vi "MDPtr DAQ Example.vi"() -> ()   [LabVIEW 2017]
uses:
  <vilib>/Utility/Data Type/Type Definitions/Data Type.ctl
  MDPtr TypeDef/MDPtr.ctl
  54395307-d518-4202-990a-94b812b105bc.vi
  9cd2cd57-26eb-46a0-897a-d177a379a7ae.vi
  4b70eac3-4565-41a8-8678-ce1595016193.vi
  <vilib>/Utility/High Resolution Relative Seconds.vi
  <vilib>/Utility/Data Type/Get Type Information.vi
  _Support/_MDPtr Validate DataFrame Type.vi
  _PolymorphicVIs/MDPtr Unpack Memory.vi
  Advanced/MDPtr DecrementCount.vi
  _PolymorphicVIs/MDPtr Pack Memory.vi
  MDPtr.lvlib
  <vilib>/measure/NI_MABase.lvlib
  _MDPtrMgr/MDPtrMgr.lvclass
  <vilib>/Utility/Data Type/NI_Data Type.lvlib
panel:
  out "time esliped?":dbl
  in  "milliseconds to wait 2":u32=1
  out "Value out":i64
  out "Queue Names":string[](array[string])
  out "time diff(s) 3":dbl
  out "time diff(s) 2":dbl
  out "time diff(s)":dbl
  in  "Fs":dbl=1000.0 format="%#_13g"
  out "# free elements in queue":i32
  out "# elements in queue":i32
  out "#queues":i32
  out "File Logging?":bool
  out "MDPtr Total Count":i64
  in  "file path":path=path "D:/MDPtr.tdms"
  out "Square":waveform(dbl)(graph)
  out "Sine":waveform(dbl)(graph)
  in  "stop":bool
  out "Copy Count":i32
  out "Common.Data Type":T1
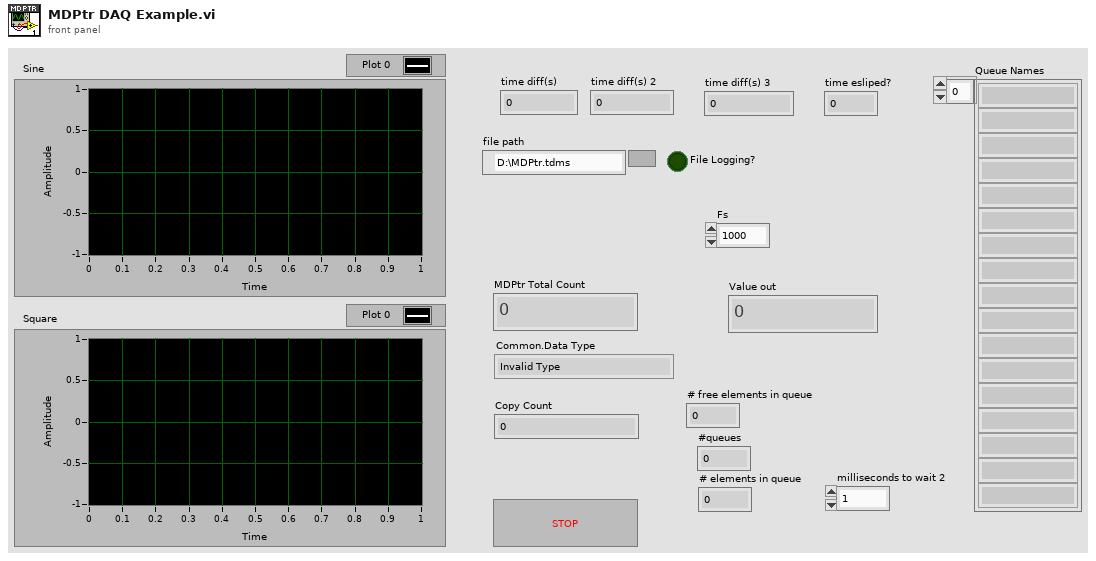
[diagram p1: front panel]
types:
  T1 = typedef "NI_Data Type.lvlib/Data Type.ctl" = enum8{"Invalid Type", "Void", "I8", "I16", "I32", "I64", "U8", "U16", "U32", "U64", "Single Float", "Double Float", "Extended Float", "Single Complex", "Double Complex", "Extended Complex", "Enum U8", "Enum U16", "Enum U32", "Enum U64", "Single Float With Unit", "Double Float With Unit", "Extended Float With Unit", "Single Complex with Unit", "Double Complex with Unit", "Extended Complex with Unit", "Boolean", "String", "Path", "Picture", "Tag", "Array", "Cluster", "Variant", "LV Variant", "Waveform", "Timestamp", "Digital Waveform", "Digital Data", "ExpressData", "Refnum", "External Data", "VI", "Poly VI", "LabVIEW Class Instance", "Fixed Point"}
  T2 = enum16{"open", "open or create", "create or replace", "create", "open (read-only)"}
  T3 = typedef "MDPtr.lvlib/MDPtr.ctl" = refnum<k1>
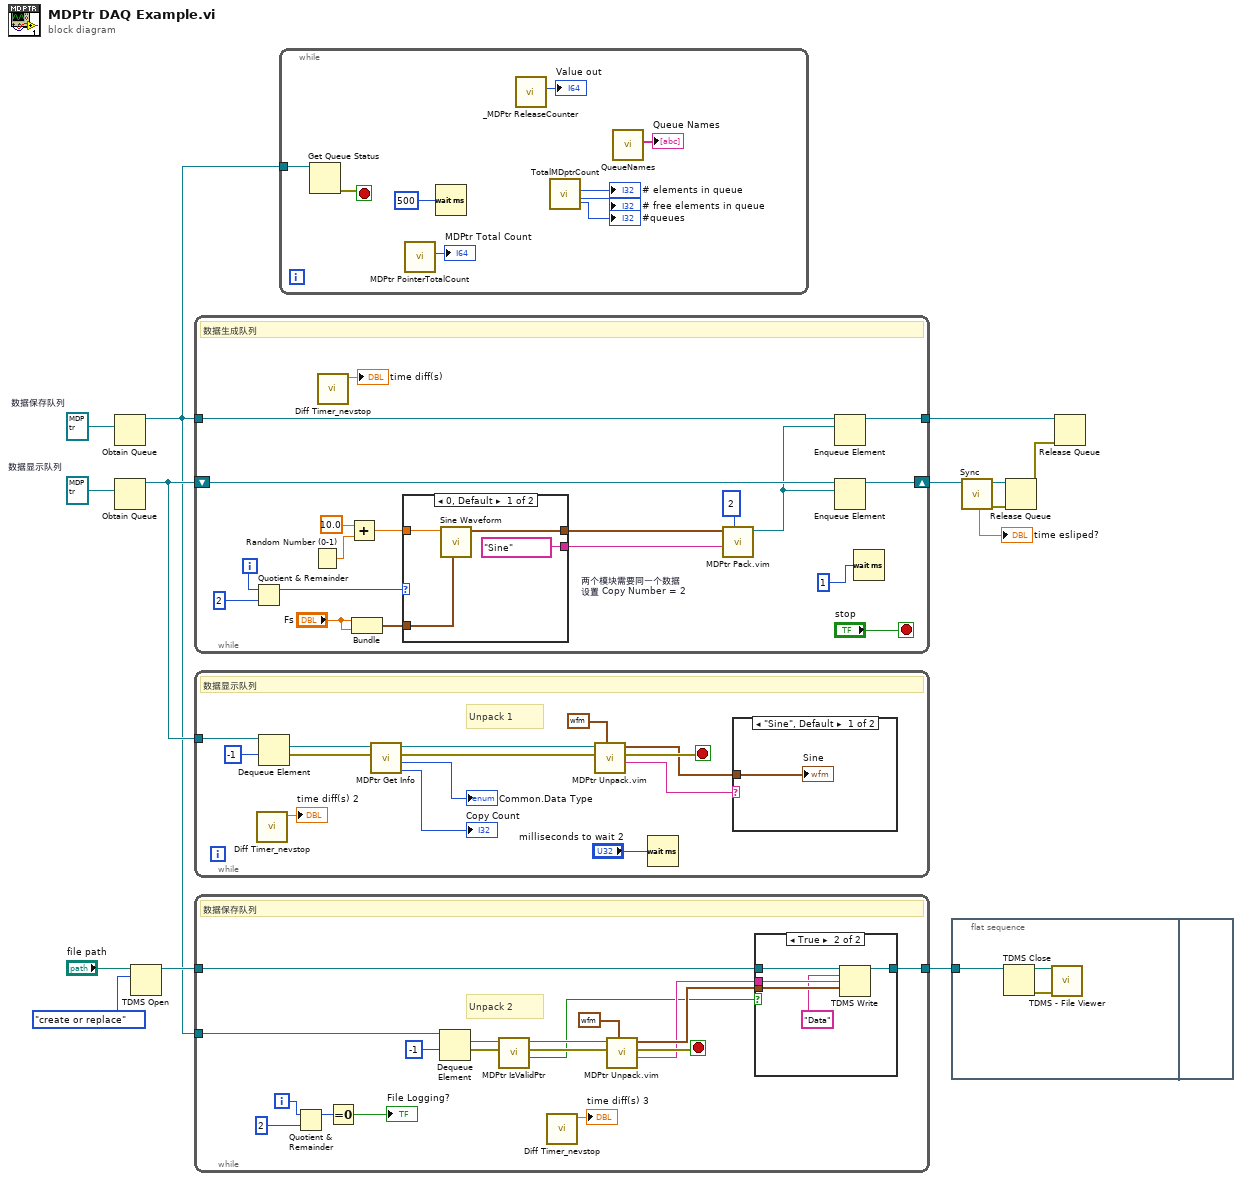
[diagram p0: block diagram]
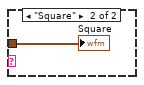
[diagram p3: hidden frame]
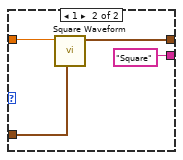
[diagram p4: hidden frame]
diagram:
  n1 = Obtain Queue "数据保存队列"(element data type=T3 refnum ("MDPtr")) -> (queue out=w4:refnum<queue>)  [unwired: 4 in, 2 out]
  n2 = Obtain Queue "数据显示队列"(element data type=T3 refnum ("MDPtr")) -> (queue out=w10:refnum<queue>)  [unwired: 4 in, 2 out]
  n3 = TDMS Open(10:T2."create or replace" ("operation (0:open)"), 11:"file path") -> (3:w8:refnum<k34>)  [unwired: 5 in, 1 out]
  n4 = while {
    shift-right: [w31] -> w5
    shift-left: w10 -> [w32]
    tunnel: w4 -> [w20]
    tunnel: [w19] -> w6
    i -> [w29]
    stop <- "stop" stop-if-true
    w21 = 2  # 两个模块需要同一个数据 设置 Copy Number = 2
    # "数据生成队列"
    n5 = Quotient & Remainder(x=w29, y=2) -> (x-y*floor(x/y)=w27:i32)  [unwired: 1 out]
    n6 = Random Number (0-1)() -> (number: 0 to 1=w23:dbl)
    n7 = call <userlib>:"Diff Timer_nevstop.vi"() -> ("time diff(s)"=→"time diff(s)":dbl)  [unwired: 10 in, 1 out]
    n8 = Add(x=10.0 ("frequency"), y=w23) -> (x+y=w22:dbl)
    n9 = Bundle("Fs"="Fs", "Fs"="Fs") -> (w15:cluster{"Fs":dbl, "Fs":dbl})  [unwired: 1 in]
    n10 = case shown="0, Default" w27 {
      tunnel: [w36 w40] -> w17
      tunnel: ["Sine" ("String Attribute") "Square" ("String Attribute")] -> w26
      tunnel: w22 -> [w34 w38]
      tunnel: w15 -> [w33 w37]
      frame 0, Default {
        n11 = call <vilib>:"Sine Waveform.vi"("sampling info"=w33, "frequency"=w34) -> ("signal out"=w36:waveform(dbl))  [unwired: 8 in, 1 out]
      }
      frame 1 {
        n12 = call <vilib>:"Square Waveform.vi"("sampling info"=w37, "frequency"=w38) -> ("signal out"=w40:waveform(dbl))  [unwired: 8 in, 1 out]
      }
    }
    n13 = call "MDPtr Pack.vim"("Copies Count(1)"=w21, "String Attribute"=w26, "Data"=w17) -> ("HexStrPtr"=w18:T3)  [unwired: 7 in, 1 out]
    n14 = Enqueue Element(queue=w20, element=w18) -> (queue out=w19:refnum<queue>)  [unwired: 2 in, 2 out]
    n15 = Enqueue Element(queue=w32, element=w18) -> (queue out=w31:refnum<queue>)  [unwired: 2 in, 2 out]
    n16 = Wait (ms)(milliseconds to wait=u32 1) -> ()  [unwired: 1 out]
  }
  n17 = while {
    tunnel: w10 -> [w54]
    stop <- w52 stop-if-true
    # "Unpack 1"
    # "数据显示队列"
    n18 = call <userlib>:"Diff Timer_nevstop.vi"() -> ("time diff(s)"=→"time diff(s) 2":dbl)  [unwired: 10 in, 1 out]
    n19 = Dequeue Element(queue=w54, timeout in ms (-1)=-1) -> (element=w44:T3, error out=w50:errorcluster)  [unwired: 1 in, 2 out]
    n20 = call "MDPtr Get Info.vi"("error in (no error)"=w50, "HexStrPtr"=w44) -> ("Copy Count"=→"Copy Count":i32, "Data Type"=→"Common.Data Type":T1, "error out"=w49:errorcluster, "HexStrPtr (dup)"=w47:T3)  [unwired: 5 in, 1 out]
    n21 = call "MDPtr Unpack.vim"("Prototype"=waveform(dbl) {"t0"=timestamp(0 s since 1904-01-01), "dt"=1.0, "Y"=[]} ("Square"), "error in (no error)"=w49, "HexStrPtr"=w47) -> ("String Attribute"=w46:string, "error out"=w52:errorcluster, "Data"=w45:waveform(dbl))  [unwired: 6 in]
    n22 = Wait (ms)(milliseconds to wait="milliseconds to wait 2") -> ()  [unwired: 1 out]
    n23 = case shown="\"Sine\", Default" w46 {
      tunnel: w45 -> [w55 w56]
      frame "Sine", Default {
        "Sine" <- w55
      }
      frame "Square" {
        "Square" <- w56
      }
    }
  }
  n24 = while {
    tunnel: w4 -> [w74]
    tunnel: [w69] -> w9
    tunnel: w8 -> [w70]
    i -> [w61]
    stop <- w72 stop-if-true
    # "Unpack 2"
    # "数据保存队列"
    n25 = Quotient & Remainder(x=w61, y=2) -> (x-y*floor(x/y)=w60:i32)  [unwired: 1 out]
    n26 = Equal To 0?(x=w60) -> (x = 0?=→"File Logging?":bool)
    n27 = Dequeue Element(queue=w74, timeout in ms (-1)=-1) -> (element=w71:T3, error out=w64:errorcluster)  [unwired: 1 in, 2 out]
    n28 = call "MDPtr IsValidPtr.vi"("error in (no error)"=w64, "HexStrPtr"=w71) -> ("Valid MDPtr?"=w63:bool, "error out"=w65:errorcluster, "HexStrPtr (dup)"=w66:T3)  [unwired: 6 in]
    n29 = call <userlib>:"Diff Timer_nevstop.vi"() -> ("time diff(s)"=→"time diff(s) 3":dbl)  [unwired: 10 in, 1 out]
    n30 = call "MDPtr Unpack.vim"("Prototype"=waveform(dbl) {"t0"=timestamp(0 s since 1904-01-01), "dt"=1.0, "Y"=[]} ("Square"), "error in (no error)"=w65, "HexStrPtr"=w66) -> ("String Attribute"=w67:string, "error out"=w72:errorcluster, "Data"=w68:waveform(dbl))  [unwired: 6 in]
    n31 = case shown="True" w63 {
      tunnel: w70 -> [w75 w80]
      tunnel: [w75 w79] -> w69
      tunnel: w68 -> [_ w78]
      tunnel: w67 -> [_ w77]
      frame False {
      }
      frame True {
        n32 = TDMS Write(0:w80, 5:"Data" ("group name in (Untitled)"), 7:w77, 9:w78) -> (4:w79:refnum<k34>)  [unwired: 2 in, 3 out]
      }
    }
  }
  n33 = while {
    tunnel: w4 -> [w89]
    stop <- w88 stop-if-true
    n34 = Get Queue Status(queue=w89) -> (error out=w88:errorcluster)  [unwired: 2 in, 7 out]
    n35 = call "MDPtr PointerTotalCount.vi"() -> ("MDPtr Total Count"=→"MDPtr Total Count":i64)  [unwired: 10 in, 1 out]
    n36 = Wait (ms)(milliseconds to wait=u32 500) -> ()  [unwired: 1 out]
    n37 = call "_MDPtr ReleaseCounter.vi"() -> ("Value out"=→"Value out":i64)  [unwired: 10 in, 1 out]
    n38 = call "TotalMDptrCount.vi"() -> ("# free elements in queue"=→"# free elements in queue":i32, "# elements in queue"=→"# elements in queue":i32, "#queues"=→"#queues":i32)  [unwired: 8 in, 1 out]
    n39 = call "QueueNames.vi"() -> ("Queue Names"=→"Queue Names":string[])  [unwired: 10 in, 1 out]
  }
  n40 = flat-sequence {
    tunnel: w9 -> [w92]
    frame #0 {
      n41 = TDMS Close(11:w92) -> (0:w91:errorcluster, 3:w90:path)  [unwired: 1 in]
      n42 = call <vilib>:"TDMS - File Viewer.vi"("error in (no error)"=w91, "file path"=w90) -> ()  [unwired: 4 in, 2 out]
    }
    frame #1 {
    }
  }
  n43 = call "Sync.vi"() -> ("error out"=w2:errorcluster, "time esliped?"=→"time esliped?":dbl)  [unwired: 9 in, 1 out]
  n44 = Release Queue(queue=w5, error in (no error)=w2) -> (error out=w3:errorcluster)  [unwired: 1 in, 2 out]
  n45 = Release Queue(queue=w6, error in (no error)=w3) -> ()  [unwired: 1 in, 3 out]
